vi "Get AccessPDO.vi"(8 "Error In":errorcluster, 11 "reference in":refnum<class "OD Entry.lvclass">) -> (0 "Error Out":errorcluster, 2 "Access PDO":T1, 3 "reference out":refnum<class "OD Entry.lvclass">)   [LabVIEW 2019, in "Electronic Datasheet.lvlib" / "OD Entry.lvclass"]
uses:
  OD Entry.lvclass
  PDO Mapping Type.ctl
  Electronic Datasheet.lvlib
  ddff5416-2aef-4ee3-b40a-6116385272f5.vi
  Access PDO.ctl
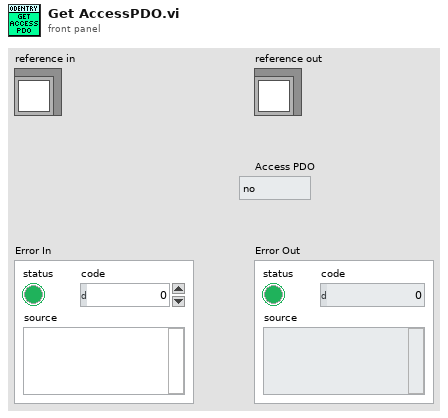
[diagram p1: front panel]
types:
  T1 = typedef "Electronic Datasheet.lvlib/Access PDO.ctl" = enum16{"no", "TPDO", "RPDO", "TPDO & RPDO"}
  T2 = enum16{"ro", "wo", "rw", "rwr", "rww", "const", "UNKNOWN"}
  T3 = typedef "Electronic Datasheet.lvlib/PDO Mapping Type.ctl" = enum16{"no", "optional", "RPDO", "TPDO", "UNKNOWN"}
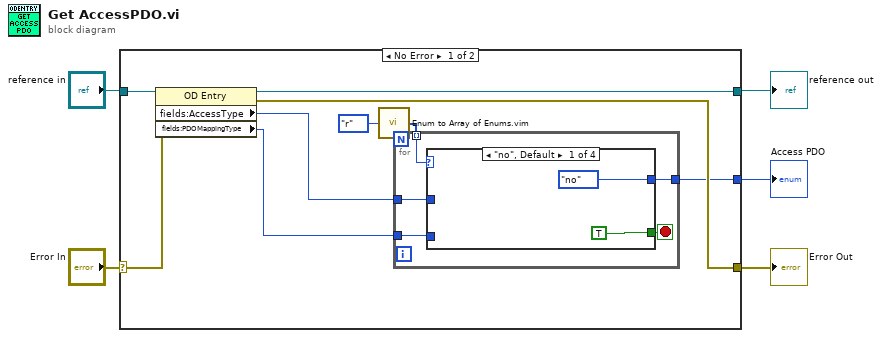
[diagram p0: block diagram]
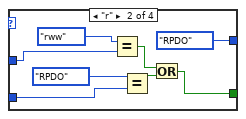
[diagram p2: hidden frame]
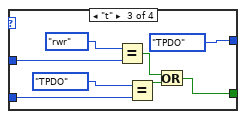
[diagram p3: hidden frame]
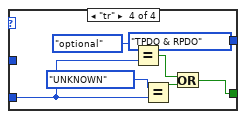
[diagram p4: hidden frame]
diagram:
  n1 = case shown="No Error" "Error In" {
    selector: "Error In" -> [w14 w46]
    tunnel: [w13 w46] -> w4
    tunnel: [w11 w45] -> w2
    tunnel: "reference in" -> [w12 w45]
    tunnel: [w6 _] -> w1
    frame No Error {
      n2 = property class="OD Entry"(reference=w12, error in=w14) -> (reference out=w11:refnum<class "OD Entry.lvclass">, error out=w13:errorcluster, "fields:AccessType"=w9:T2, "fields:PDOMappingType"=w8:T3)
      n3 = call "Enum to Array of Enums.vim"("enum"=enum16{"r", "t", "tr", "no"}."r") -> ("array of enums"=w10:enum16{"r", "t", "tr", "no"}[])
      n4 = for {
        tunnel: w10 -> [w19] mode=indexing
        tunnel: w9 -> [w18]
        tunnel: w8 -> [w17]
        tunnel: [w15] -> w6
        stop <- w16 stop-if-true
        n5 = case shown="\"no\", Default" w19 {
          tunnel: w18 -> [_ w23 w34 _]
          tunnel: w17 -> [_ w24 w32 w40]
          tunnel: [TRUE w27 w35 w42] -> w16
          tunnel: [Access_PDO."no" ("Access PDO") Access_PDO."RPDO" ("Access PDO") Access_PDO."TPDO" ("Access PDO") Access_PDO."TPDO & RPDO" ("Access PDO")] -> w15
          frame "no", Default {
          }
          frame "r" {
            n6 = Equal?(x=T2."rww" ("y"), y=w23) -> (x = y?=w29:bool)
            n7 = Equal?(x=PDO_Mapping_Type."RPDO" ("y"), y=w24) -> (x = y?=w28:bool)
            n8 = Or(x=w29, y=w28) -> (x .or. y?=w27:bool)
          }
          frame "t" {
            n9 = Equal?(x=T2."rwr" ("y"), y=w34) -> (x = y?=w37:bool)
            n10 = Equal?(x=PDO_Mapping_Type."TPDO" ("y"), y=w32) -> (x = y?=w36:bool)
            n11 = Or(x=w37, y=w36) -> (x .or. y?=w35:bool)
          }
          frame "tr" {
            n12 = Equal?(x=PDO_Mapping_Type."optional", y=w40) -> (x = y?=w44:bool)
            n13 = Equal?(x=PDO_Mapping_Type."UNKNOWN", y=w40) -> (x = y?=w43:bool)
            n14 = Or(x=w44, y=w43) -> (x .or. y?=w42:bool)
          }
        }
      }
    }
    frame Error {
    }
  }
  "Error Out" <- w4
  "reference out" <- w2
  "Access PDO" <- w1
